vi "DIELECdll.vi"(8 "error in (no error)":errorcluster, 9 "z":dbl[](array[numeric]), 10 "D":dbl, 11 "t":dbl) -> (0 "error out":errorcluster, 3 "de":dbl)   [LabVIEW 2016]
doc: "subroutine DIELECdll(t, D, z, de)\n\nCompute dielectric constant as a function of temperature, density, and composition.\n\nINPUTS:\nt --Temperature [K]\nD -- Molar density [mol/L]\nz -- Composition (array of mole fractions)\n\nOUTPUTS:\nde -- Dielectric constant"
uses:
  REFPROP.DLL
panel:
  # "REFPROP-DIELECdll.vi"
  # "void  DIELECdll(double *t, double *D, double *z, double *de)"
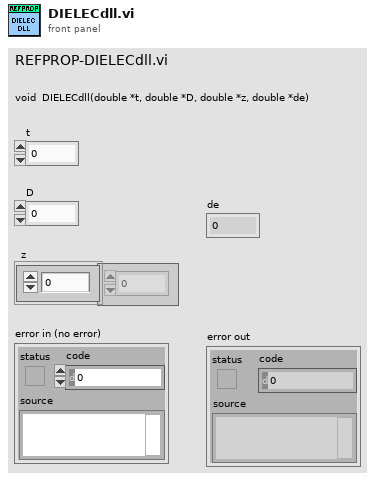
[diagram p1: front panel]
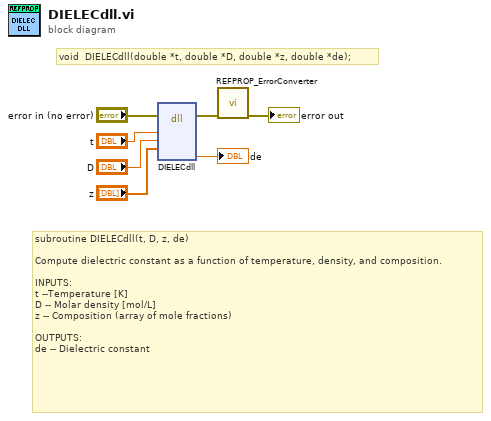
[diagram p0: block diagram]
diagram:
  # "void  DIELECdll(double *t, double *D, double *z, double *de);"
  # "subroutine DIELECdll(t, D, z, de)\n\nCompute dielectric constant as a function of temperature, density, and composition.\n\nINPUTS:\nt --Temperature [K]\nD -- Molar density [mol/L]\nz -- Composition (array of mole fractions)\n\nOUTPUTS:\nde -- Dielectric constant"
  n1 = dll-call lib="S:/009 - Testing/02 - Performance Testing/REFPROP/REFPROP.*" fn="DIELECdll"(error in="error in (no error)", "t"="t", "D"="D", "z"="z") -> (error out=w3:errorcluster, "de"=→"de":dbl)  [unwired: 7 in, 1 out]
  n2 = call "REFPROP_ErrorConverter.vi"("error in (no error)"=w3) -> ("error out"=→"error out":errorcluster)  [unwired: 10 in]
